vi "Configure Output Pon State.vi"(8 "error in":errorcluster, 10 "State":u16(ring) items=["RST", "LAST", "LAST_OFF"], 11 "VISA resource name":refnum<visa-resource-name>) -> (0 "error out":errorcluster, 3 "VISA resource name out":refnum<visa-resource-name>)   [LabVIEW 2015, in "IT-M3900C.lvlib"]
doc: "This command is used to control some parameters and output state: on or off.\n<b>State</b>\n0: RST: default value, indicating the initial value displayed when the instrument is powered on.Detailed parameters are described in *RST.\n1: LAST: represents the parameter Settings and output state displayed by the instrument when it is powered up next time.\n2: LAST_OFF: indicates that the parameters displayed when the instrument is powered up next time are set to the parameters set this time, and the output state is Off."
uses:
  <instrlib>/IT-M3900C/IT-M3900C.lvlib
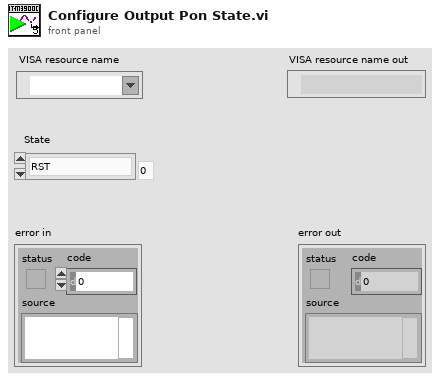
[diagram p1: front panel]
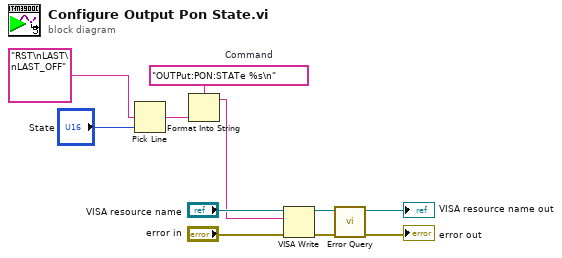
[diagram p0: block diagram]
diagram:
  w5 = "OUTPut:PON:STATe %s\n"  # Command
  n1 = Pick Line(multi-line string="RST\nLAST\nLAST_OFF", line index="State") -> (output string=w1:string)  [unwired: 1 in]
  n2 = Format Into String(format string=w5, w1) -> (resulting string=w4:string)  [unwired: 2 in, 1 out]
  n3 = VISA Write(VISA resource name="VISA resource name", write buffer=w4, error in (no error)="error in") -> (VISA resource name out=w8:refnum<visa-resource-name>, error out=w9:errorcluster)  [unwired: 1 out]
  n4 = call <instrlib>:"Error Query.vi"("error in"=w9, "VISA resource name"=w8) -> ("error out"=→"error out":errorcluster, "VISA resource name out"=→"VISA resource name out":refnum<visa-resource-name>)  [unwired: 6 in, 2 out]
